vi "AR-Timer-2.vi"(7 "Action":enum16{"Reset", "Start"}(ring), 8 "error in":errorcluster, 10 "Reset":bool, 11 "Target (mS)":u32) -> (0 "error out":errorcluster, 2 "Time Elapsed":bool, 3 "Loop time (ms)":u32)   [LabVIEW 2021]
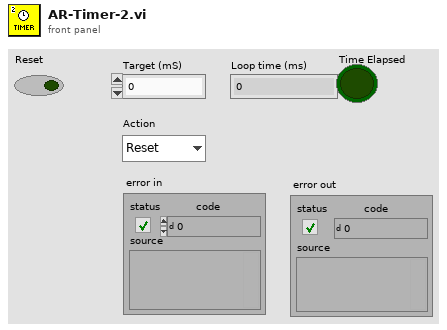
[diagram p1: front panel]
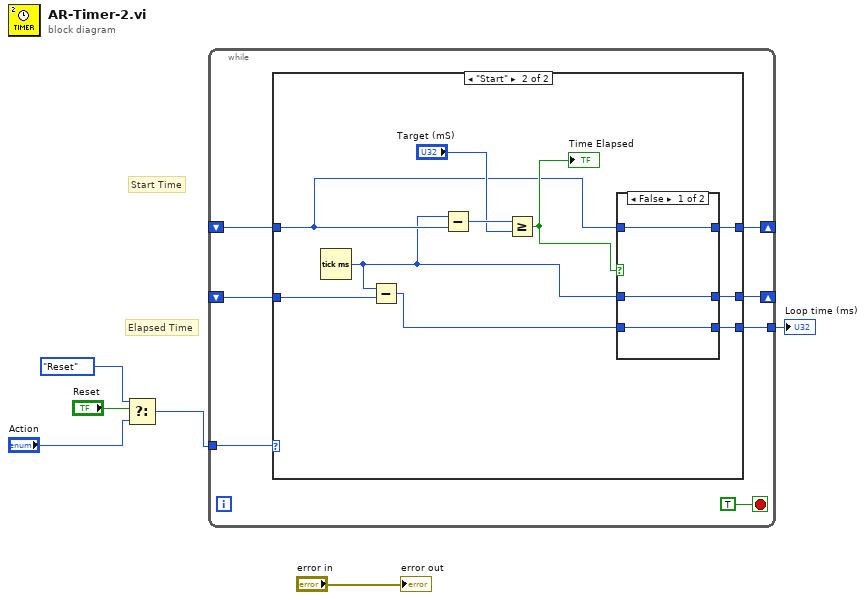
[diagram p0: block diagram]
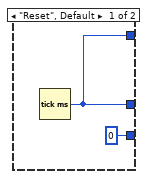
[diagram p2: hidden frame]
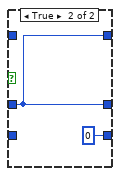
[diagram p3: hidden frame]
diagram:
  # "Elapsed Time"
  # "Start Time"
  n1 = Select(t=enum16{"Reset", "Start"}."Reset" ("Action"), s="Reset", f="Action") -> (s? t:f=w1:enum16{"Reset", "Start"})
  n2 = while {
    shift-right: [w10] -> _
    shift-left: _ -> [w12]
    tunnel: [w9] -> w6
    shift-right: [w8] -> _
    shift-left: _ -> [w7]
    tunnel: w1 -> [w11]
    stop <- TRUE stop-if-true
    n3 = case shown="\"Start\"" w11 {
      tunnel: w12 -> [_ w25]
      tunnel: [w15 w18] -> w10
      tunnel: [u32 0 w16] -> w9
      tunnel: [w15 w20] -> w8
      tunnel: w7 -> [_ w21]
      frame "Reset", Default {
        n4 = Tick Count (ms)() -> (millisecond timer value=w15:u32)
      }
      frame "Start" {
        n5 = Tick Count (ms)() -> (millisecond timer value=w19:u32)
        n6 = Subtract(x=w19, y=w25) -> (x-y=w17:u32)
        n7 = Subtract(x=w19, y=w21) -> (x-y=w24:u32)
        n8 = Greater Or Equal?(x=w24, y="Target (mS)") -> (x >= y?=w22:bool)
        "Time Elapsed" <- w22
        n9 = case shown="False" w22 {
          tunnel: w21 -> [w28 _]
          tunnel: [w28 w30] -> w20
          tunnel: w19 -> [w27 w30]
          tunnel: [w27 w30] -> w18
          tunnel: w17 -> [w26 _]
          tunnel: [w26 u32 0] -> w16
          frame False {
          }
          frame True {
          }
        }
      }
    }
  }
  "Loop time (ms)" <- w6
  "error out" <- "error in"
